vi "Get Full Help.vi"(8 "error in (no error)":errorcluster, 11 "Install in":refnum<class "Install.lvclass">) -> (0 "error out":errorcluster, 2 "Full Help":string, 3 "Install out":refnum<class "Install.lvclass">)   [LabVIEW 2020, in "Install.lvlib" / "Install.lvclass"]
uses:
  Install.lvclass
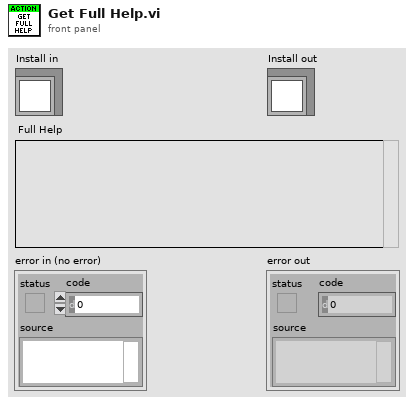
[diagram p1: front panel]
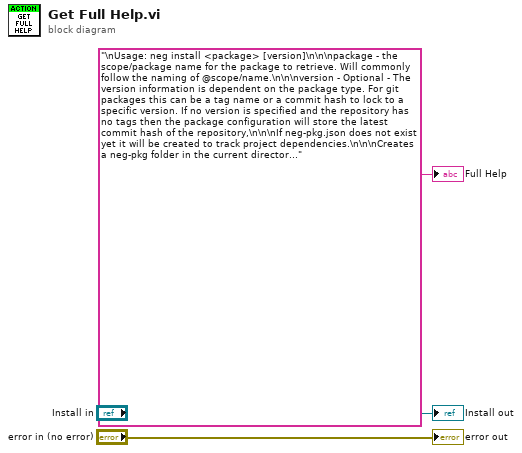
[diagram p0: block diagram]
diagram:
  "error out" <- "error in (no error)"
  "Install out" <- "Install in"
  "Full Help" <- "\nUsage: neg install <package> [version]\n\n\npackage - the scope/package name for the package to retrieve. Will commonly follow the naming of @scope/name.\n\n\nversion - Optional - The version information is dependent on the package type. For git packages this can be a tag name or a commit hash to lock to a specific version. If no version is specified and the repository has no tags then the package configuration will store the latest commit hash of the repository,\n\n\nIf neg-pkg.json does not exist yet it will be created to track project dependencies.\n\n\nCreates a neg-pkg folder in the current directory to clone packages to if it does not already exist. After installation, dependencies will manually need to be added to relevant project(s)." ("Full Help")
